vi "MoveRef.vi"(8 "error in":errorcluster, 9 "Axis":i32, 10 "Position":dbl, 11 "VISA resource":refnum<visa-resource-name>) -> (0 "error out":errorcluster)   [LabVIEW 2014, in "GRBLMotionCore.lvlib"]
uses:
  <instrlib>/GRBL/GRBLMotionCore.lvlib
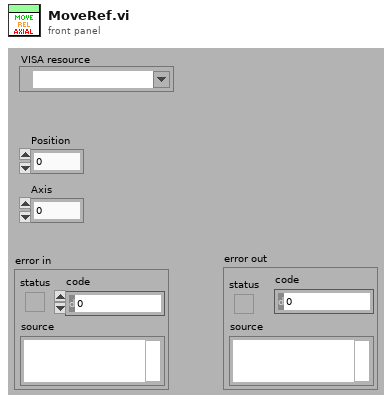
[diagram p1: front panel]
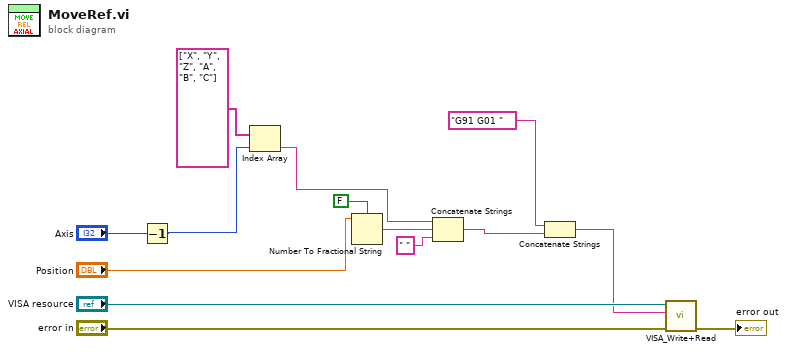
[diagram p0: block diagram]
diagram:
  n1 = Decrement(x="Axis") -> (x-1=w2:i32)
  n2 = Index Array(array=string[] ["X", "Y", "Z", "A", "B", "C"], index=w2) -> (element=w7:string)
  n3 = Number To Fractional String(use system decimal point (T)=FALSE, number="Position") -> (F-format string=w9:string)  [unwired: 2 in]
  n4 = Concatenate Strings(w7, w9, " " ("string")) -> (w4:string)
  n5 = Concatenate Strings("G91 G01 ", w4) -> (w3:string)
  n6 = call <instrlib>:"VISA_Write+Read.vi"("error in (no error)"="error in", "Write Buffer"=w3, "VISA resource name"="VISA resource") -> ("error out"=→"error out":errorcluster)  [unwired: 6 in, 2 out]
